vi "Subscribe to Topics.vi"(8 "error in (no error)":errorcluster, 11 "message session in":refnum<class "NI Skyline Message.lvclass">) -> (0 "error out":errorcluster, 3 "message session out":refnum<class "NI Skyline Message.lvclass">)   [LabVIEW 2020]
doc: "Using a created SL Messaging session, this VI subscribes to the topics expected to be sent by the G Web UI."
uses:
  <vilib>/Skyline/Message/NI Skyline Message.lvclass
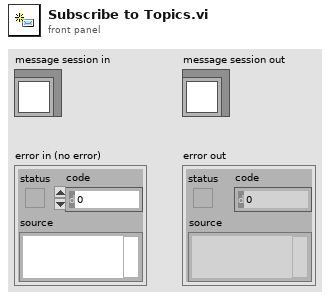
[diagram p1: front panel]
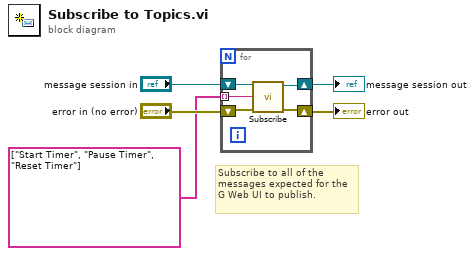
[diagram p0: block diagram]
diagram:
  # "Subscribe to all of the messages expected for the G Web UI to publish."
  n1 = for {
    tunnel: string[] ["Start Timer", "Pause Timer", "Reset Timer"] -> [w8] mode=indexing
    shift-right: [w7] -> w2
    shift-left: "message session in" -> [w10]
    shift-right: [w6] -> w1
    shift-left: "error in (no error)" -> [w9]
    n2 = call-dynamic "Subscribe.vi"("error in (no error)"=w9, "topic"=w8, "message session in"=w10) -> ("error out"=w6:errorcluster, "message session out"=w7:refnum<class "NI Skyline Message.lvclass">)  [unwired: 7 in]
  }
  "error out" <- w1
  "message session out" <- w2
